vi "BASE_I_O_Screen.vi"(8 "error in (no error)":errorcluster) -> (0 "error out":errorcluster)   [LabVIEW 2017]
doc: "This vi is for manually turn ON and OFF also monitor Output of PLCS. So this is manual screen."
uses:
  <vilib>/Utility/file.llb/Read Delimited Spreadsheet (string).vi
panel:
  in  "Tab Control":enum32{"OUTPUT", "INPUT"}(tab)
  out "OUTPUT":T1
  out "INPUT":T1
  out "CARD 8 OUTPUT":T2
  in  "Back":bool
  # "I/O Screen"
  # "INPUT"
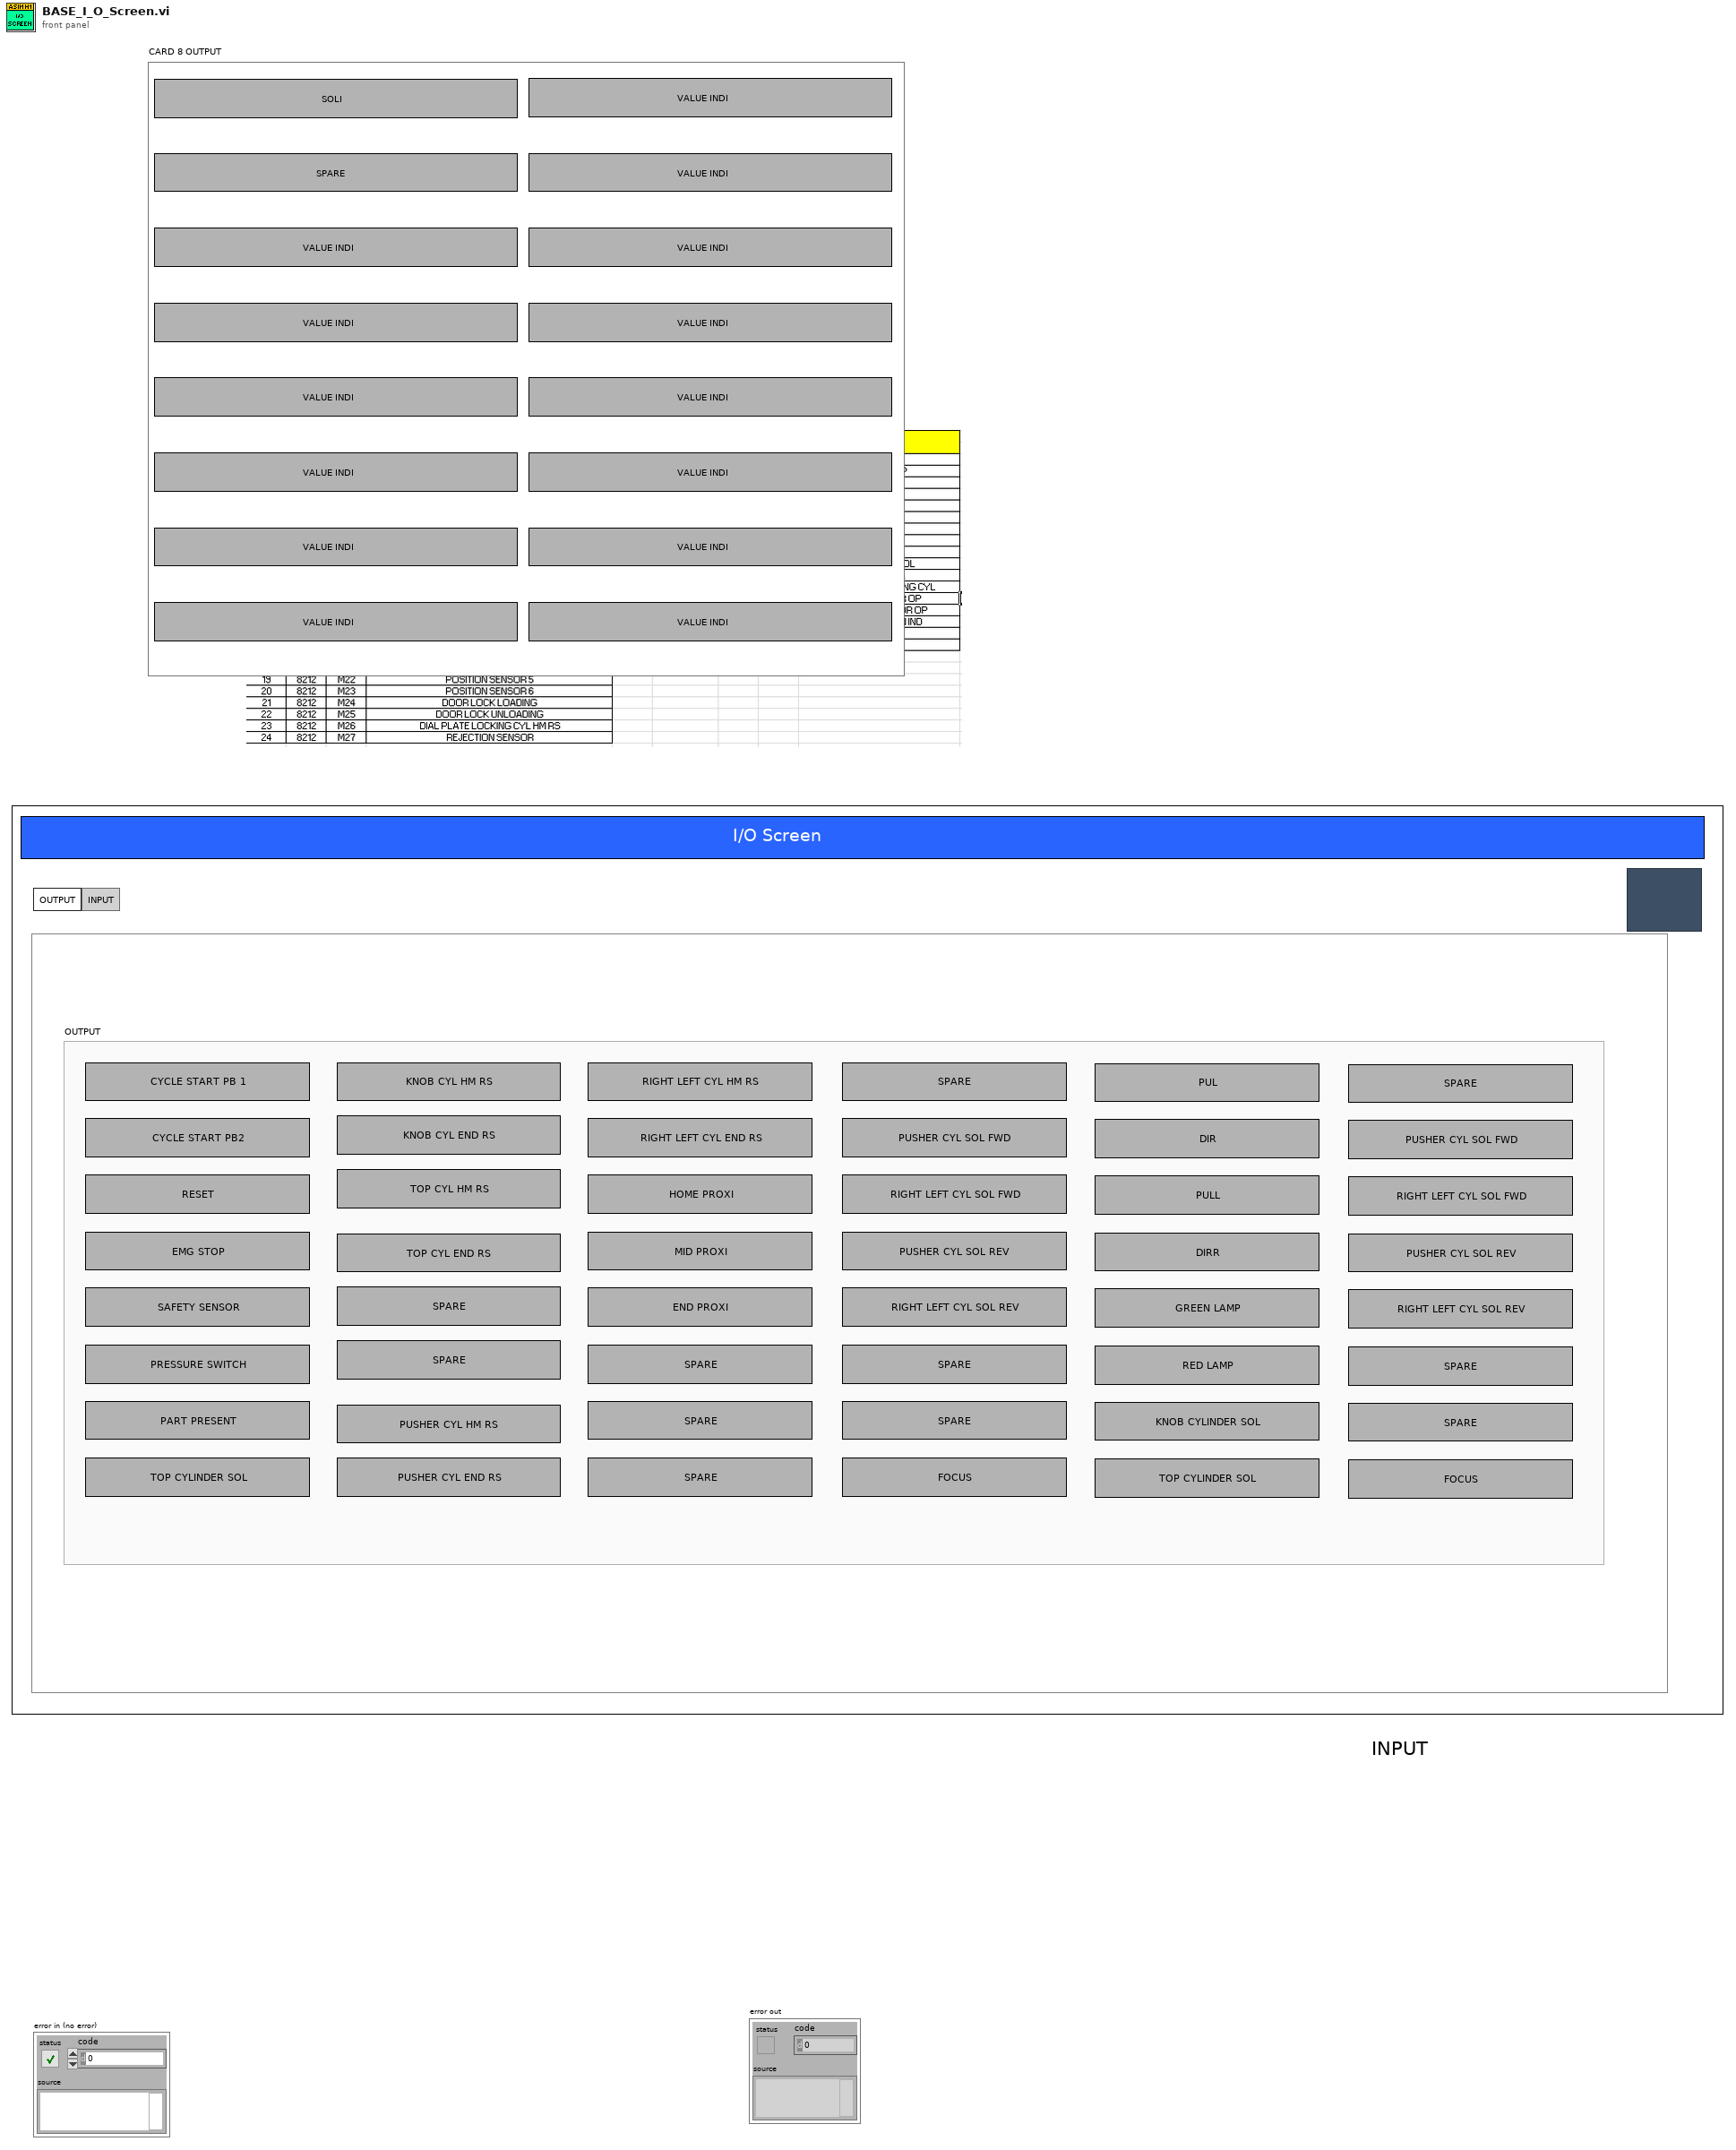
[diagram p1: front panel]
types:
  T1 = cluster{"GREEN LAMP":bool, "RED LAMP":bool, "BUZZER":bool, "PART CLAMP SOL":bool, " THREAD LOCKER ON":bool, "THREAD LOCKER OFF":bool, "PUSHER FWD SOL":bool, "UP DN CYL FWD SOL":bool, "UP DN CYL REV SOL":bool, "Y20-SPARE":bool, "Y21":bool, "Y22 2":bool, "Y22":bool, "Y23":bool, "Y25":bool, "GREEN LAMP 2":bool, "RED LAMP 2":bool, "BUZZER 2":bool, "PART CLAMP SOL 2":bool, " THREAD LOCKER ON 2":bool, "THREAD LOCKER OFF 2":bool, "PUSHER FWD SOL 2":bool, "PUSHER REV SOL 2":bool, "UP DN CYL FWD SOL 2":bool, "UP DN CYL REV SOL 2":bool, "Y20-SPARE 2":bool, "Y21 2":bool, "Y22 3":bool, "Y22 4":bool, "Y23 2":bool, "Y25 2":bool, "GREEN LAMP 3":bool, "RED LAMP 3":bool, "BUZZER 3":bool, "PART CLAMP SOL 3":bool, " THREAD LOCKER ON3":bool, "THREAD LOCKER OFF 3":bool, "PUSHER FWD SOL 3":bool, "PUSHER REV SOL 3":bool, "UP DN CYL FWD SOL 3":bool, "UP DN CYL REV SOL 3":bool, "Y20-SPARE 3":bool, "Y21 3":bool, "Y22 5":bool, "Y22 6":bool, "Y23 3":bool, "Y25 3":bool, "PUSHER REV SOL":bool}
  T2 = cluster{"8 CARD 1":bool, "8 CARD 2":bool, "8 CARD 3":bool, "8 CARD 4":bool, "8 CARD 5":bool, "8 CARD 6":bool, "8 CARD 7":bool, "8 CARD 8":bool, "8 CARD 9":bool, "8 CARD 10":bool, "8 CARD 11":bool, "8 CARD 12":bool, "8 CARD 13":bool, "8 CARD 14":bool, "8 CARD 15":bool, "8 CARD 16":bool}
  T3 = enum32{"invalid app kind", "Development System", "Run Time System", "Student Edition", "Embedded LabVIEW", "Evaluation", "Custom"}
  T4 = enum32{"Invalid", "Standard", "Closed", "Hidden", "Minimized", "Maximized"}
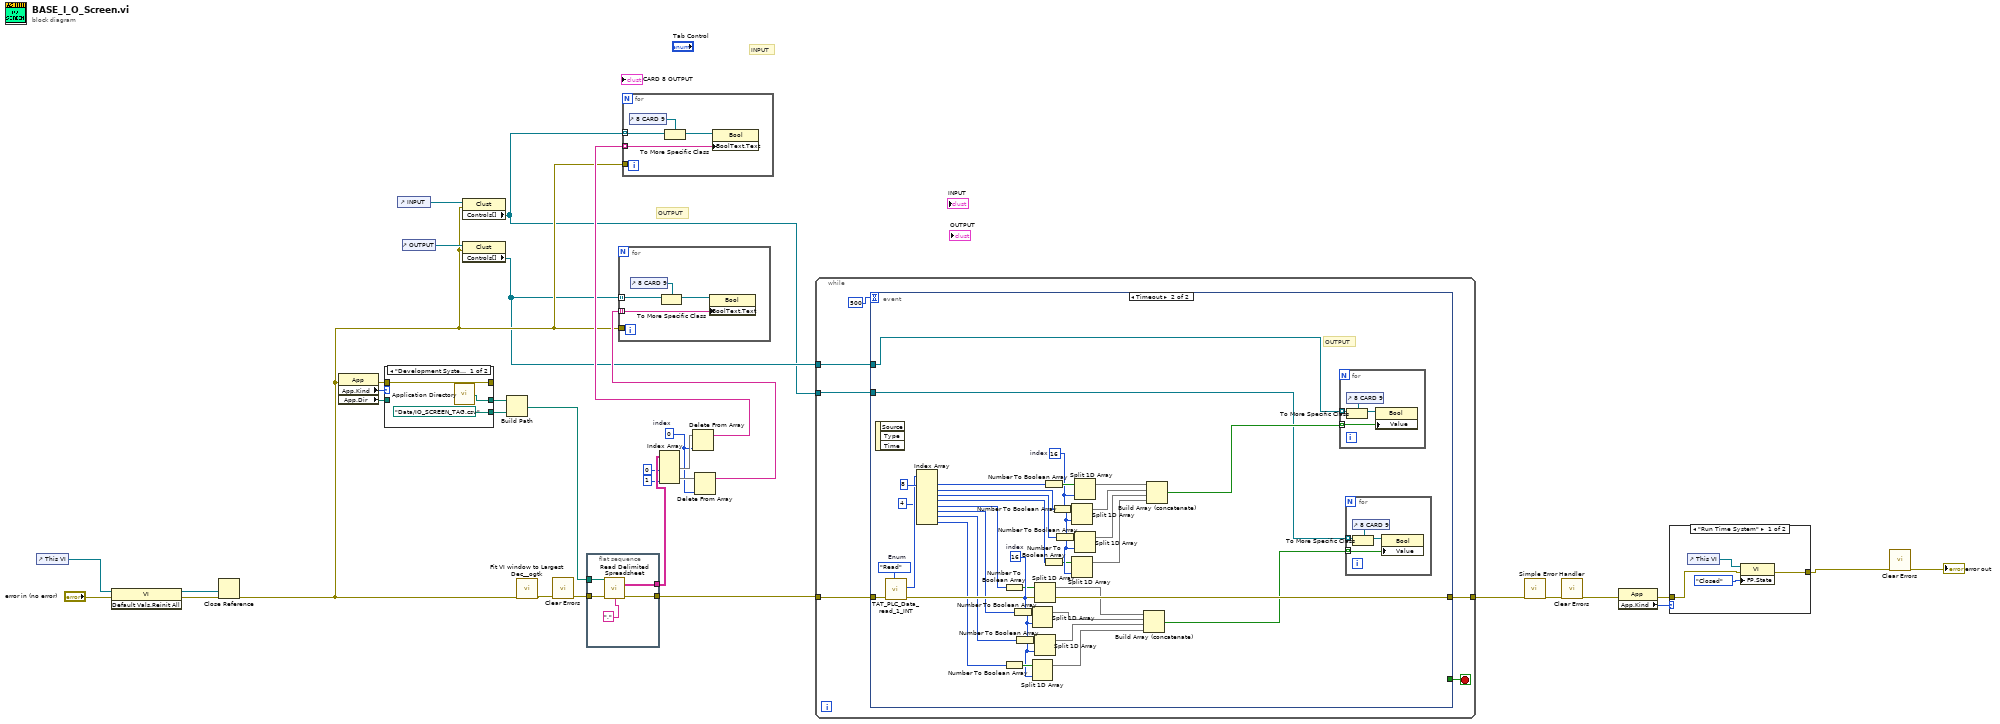
[diagram p0: block diagram]
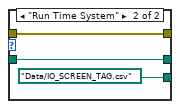
[diagram p2: hidden frame]
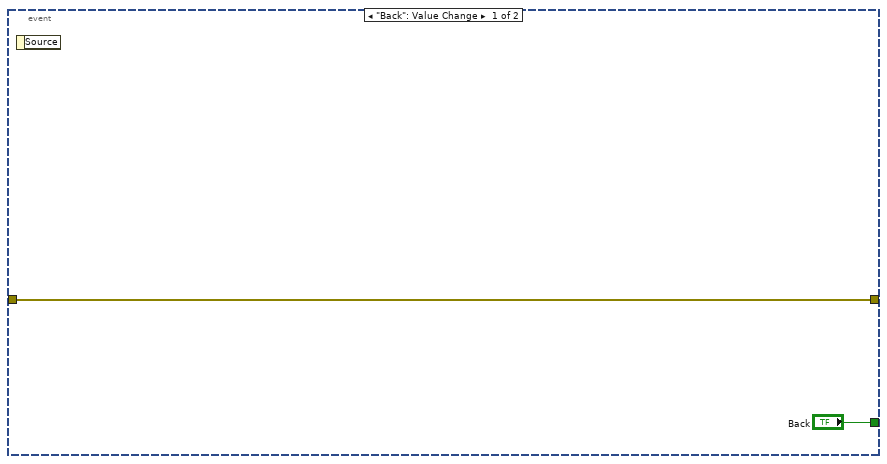
[diagram p4: hidden frame]
diagram:
  w17 = 0  # index
  # "OUTPUT"
  # "INPUT"
  n1 = control-ref of="This VI"() -> (w30:refnum<vi>)
  n2 = invoke class="VI" method="Default Vals.Reinit All"(reference=w30, error in="error in (no error)") -> (reference out=w28:refnum<vi>, error out=w27:errorcluster)  [unwired: 1 in, 1 out]
  n3 = Close Reference(reference=w28, error in (no error)=w27) -> (error out=w4:errorcluster)
  n4 = property class="App"(error in=w4) -> (error out=w12:errorcluster, "App.Kind"=w10:T3, "App.Dir"=w11:path)  [unwired: 1 in, 1 out]
  n5 = case shown="\"Development System\", Default" w10 {
    tunnel: [w36 w39] -> _
    tunnel: w12 -> [w36 w39]
    tunnel: w11 -> [_ w38]
    tunnel: [w34 w38] -> w13
    tunnel: [path "Data/IO_SCREEN_TAG.csv" path "Data/IO_SCREEN_TAG.csv"] -> w14
    frame "Development System", Default {
      n6 = call <vilib>:"Application Directory.vi"() -> ("Application Directory"=w34:path)
    }
    frame "Run Time System" {
    }
  }
  n7 = control-ref of="INPUT"() -> (w2:refnum<vi>)
  n8 = control-ref of="OUTPUT"() -> (w5:refnum<vi>)
  n9 = property on="Property Node" class="Clust"(reference=w2, error in=w4) -> ("Controls[]"=w1:refnum<vi>[])  [unwired: 2 out]
  n10 = property on="Property Node" class="Clust"(reference=w5, error in=w4) -> ("Controls[]"=w3:refnum<vi>[])  [unwired: 2 out]
  n11 = Build Path(base path=w13, name or relative path=w14) -> (appended path=w9:path)
  n12 = call <userlib>:"Fit VI window to Largest Dec__ogtk.vi"("error in (no error)"=w4) -> ("error out"=w15:errorcluster)  [unwired: 5 in, 1 out]
  n13 = call <vilib>:"Clear Errors.vi"("error in (no error)"=w15) -> ("error out"=w8:errorcluster)  [unwired: 5 in, 1 out]
  n14 = flat-sequence {
    tunnel: w8 -> [w43]
    tunnel: [w44] -> w16
    tunnel: w9 -> [w42]
    tunnel: [w40] -> w22
    frame #0 {
      n15 = call-poly <vilib>:"Read Delimited Spreadsheet.vi"("file path (dialog if empty)"=w42, "error in (no error)"=w43, "delimiter (\\t)"=",") -> ("all rows"=w40:string[][], "error out"=w44:errorcluster)  [unwired: 7 in, 4 out]
    }
  }
  n16 = Index Array(array=w22, index (col) #1=0, index (col) #2=1) -> (element #1=w19:string[], element #2=w18:string[])  [unwired: 2 in]
  n17 = Delete From Array(array=w19, index=w17) -> (array with subset deleted=w7:string[])  [unwired: 1 in, 1 out]
  n18 = for {
    tunnel: w7 -> [w46] mode=indexing
    tunnel: w1 -> [w45] mode=indexing
    tunnel: w4 -> [_]
    n19 = control-ref of="8 CARD 9"() -> (w47:refnum<vi>)
    n20 = To More Specific Class(target class=w47, reference=w45) -> (specific class reference=w48:refnum<vi>)  [unwired: 1 in, 1 out]
    n21 = property on="Property Node" class="Bool"(reference=w48, "BoolText.Text"=w46) -> ()  [unwired: 1 in, 2 out]
  }
  n22 = Delete From Array(array=w18, index=w17) -> (array with subset deleted=w6:string[])  [unwired: 1 in, 1 out]
  n23 = for {
    tunnel: w6 -> [w50] mode=indexing
    tunnel: w3 -> [w49] mode=indexing
    tunnel: w4 -> [_]
    n24 = control-ref of="8 CARD 9"() -> (w51:refnum<vi>)
    n25 = To More Specific Class(target class=w51, reference=w49) -> (specific class reference=w52:refnum<vi>)  [unwired: 1 in, 1 out]
    n26 = property on="Property Node" class="Bool"(reference=w52, "BoolText.Text"=w50) -> ()  [unwired: 1 in, 2 out]
  }
  n27 = while {
    tunnel: w16 -> [w58]
    tunnel: [w57] -> w32
    tunnel: w3 -> [w54]
    tunnel: w1 -> [w53]
    stop <- w56 stop-if-true
    n28 = event shown="[1] Timeout" {
      selector: _ -> [_ _]
      dyn-events: _ -> [_ _]
      timeout: 500 -> [_ _]
      tunnel: w58 -> [w59 w83]
      tunnel: [w59 w82] -> w57
      tunnel: ["Back" _] -> w56
      tunnel: w54 -> [_ w79]
      tunnel: w53 -> [_ w76]
      event "Back": Value Change {
        n29 = event-data() -> ()  [unwired: 1 in, 1 out]
      }
      event Timeout {
        w70 = 16  # index
        w84 = enum16{"Read", "Write"}."Read"  # Enum
        w90 = 16  # index
        # "OUTPUT"
        n30 = event-data() -> ()  [unwired: 1 in, 3 out]
        n31 = call "TAT_PLC_Data_read_1_INT.vi"("Enum"=w84, "error in (no error)"=w83) -> ("error out"=w82:errorcluster, "Array 2"=w81:u16[])  [unwired: 8 in]
        n32 = Index Array(array=w81, index #1=8, index #5=4) -> (element #1=w96:u16, element #2=w92:u16, element #3=w89:u16, element #4=w88:u16, element #5=w65:u16, element #6=w64:u16, element #7=w63:u16, element #8=w62:u16)  [unwired: 6 in]
        n33 = Number To Boolean Array(number=w65) -> (Boolean array=w67:bool[])
        n34 = Number To Boolean Array(number=w62) -> (Boolean array=w71:bool[])
        n35 = Number To Boolean Array(number=w64) -> (Boolean array=w68:bool[])
        n36 = Number To Boolean Array(number=w63) -> (Boolean array=w69:bool[])
        n37 = Split 1D Array(array=w68, index=w70) -> (first subarray=w75:bool[])  [unwired: 1 out]
        n38 = Split 1D Array(array=w71, index=w70) -> (first subarray=w73:bool[])  [unwired: 1 out]
        n39 = Split 1D Array(array=w67, index=w70) -> (first subarray=w74:bool[])  [unwired: 1 out]
        n40 = Split 1D Array(array=w69, index=w70) -> (first subarray=w72:bool[])  [unwired: 1 out]
        n41 = Number To Boolean Array(number=w96) -> (Boolean array=w95:bool[])
        n42 = Number To Boolean Array(number=w88) -> (Boolean array=w87:bool[])
        n43 = Number To Boolean Array(number=w92) -> (Boolean array=w93:bool[])
        n44 = Number To Boolean Array(number=w89) -> (Boolean array=w91:bool[])
        n45 = Split 1D Array(array=w93, index=w90) -> (first subarray=w77:bool[])  [unwired: 1 out]
        n46 = Split 1D Array(array=w87, index=w90) -> (first subarray=w85:bool[])  [unwired: 1 out]
        n47 = Split 1D Array(array=w95, index=w90) -> (first subarray=w78:bool[])  [unwired: 1 out]
        n48 = Split 1D Array(array=w91, index=w90) -> (first subarray=w86:bool[])  [unwired: 1 out]
        n49 = Build Array (concatenate)(w74, w75, w72, w73) -> (w61:bool[])
        n50 = Build Array (concatenate)(w78, w77, w86, w85) -> (w80:bool[])
        n51 = for {
          tunnel: w80 -> [w102] mode=indexing
          tunnel: w79 -> [w101] mode=indexing
          n52 = control-ref of="8 CARD 9"() -> (w103:refnum<vi>)
          n53 = To More Specific Class(target class=w103, reference=w101) -> (specific class reference=w104:refnum<vi>)  [unwired: 1 in, 1 out]
          n54 = property on="Property Node" class="Bool"(reference=w104, "Value"=w102) -> ()  [unwired: 1 in, 2 out]
        }
        n55 = for {
          tunnel: w76 -> [w98] mode=indexing
          tunnel: w61 -> [w97] mode=indexing
          n56 = control-ref of="8 CARD 9"() -> (w99:refnum<vi>)
          n57 = To More Specific Class(target class=w99, reference=w98) -> (specific class reference=w100:refnum<vi>)  [unwired: 1 in, 1 out]
          n58 = property on="Property Node" class="Bool"(reference=w100, "Value"=w97) -> ()  [unwired: 1 in, 2 out]
        }
      }
    }
  }
  n59 = call <vilib>:"Simple Error Handler.vi"("error in (no error)"=w32) -> ("error out"=w26:errorcluster)  [unwired: 4 in, 4 out]
  n60 = call <vilib>:"Clear Errors.vi"("error in (no error)"=w26) -> ("error out"=w23:errorcluster)  [unwired: 5 in, 1 out]
  n61 = property class="App"(error in=w23) -> (error out=w24:errorcluster, "App.Kind"=w25:T3)  [unwired: 1 in, 1 out]
  n62 = case shown="\"Run Time System\"" w25 {
    tunnel: w24 -> [w106 w109]
    tunnel: [w105 w109] -> w31
    frame "Run Time System" {
      n63 = control-ref of="This VI"() -> (w108:refnum<vi>)
      n64 = property class="VI"(reference=w108, error in=w106, "FP.State"=T4."Closed" ("Front Panel Window:State")) -> (error out=w105:errorcluster)  [unwired: 1 out]
    }
    frame "Development System", Default {
    }
  }
  n65 = call <vilib>:"Clear Errors.vi"("error in (no error)"=w31) -> ("error out"=→"error out":errorcluster)  [unwired: 5 in, 1 out]
